vi "getScanValues.vi"(8 "error in (no error)":errorcluster, 11 "ScanCreator in":refnum<class "ScanCreator.lvclass">) -> (0 "error out":errorcluster, 1 "stop":dbl, 2 "start":dbl, 3 "ScanCreator out":refnum<class "ScanCreator.lvclass">, 4 "step":i16)   [LabVIEW 2009, in "Views.lvlib" / "ScriptEditor.lvlib" / "ScanCreator.lvclass"]
uses:
  ScanCreator.lvclass
  ScanCreator.lvclass/ScanCreator.ctl
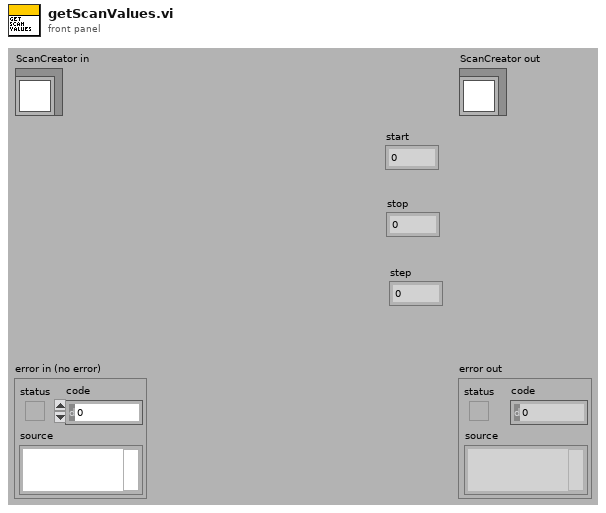
[diagram p1: front panel]
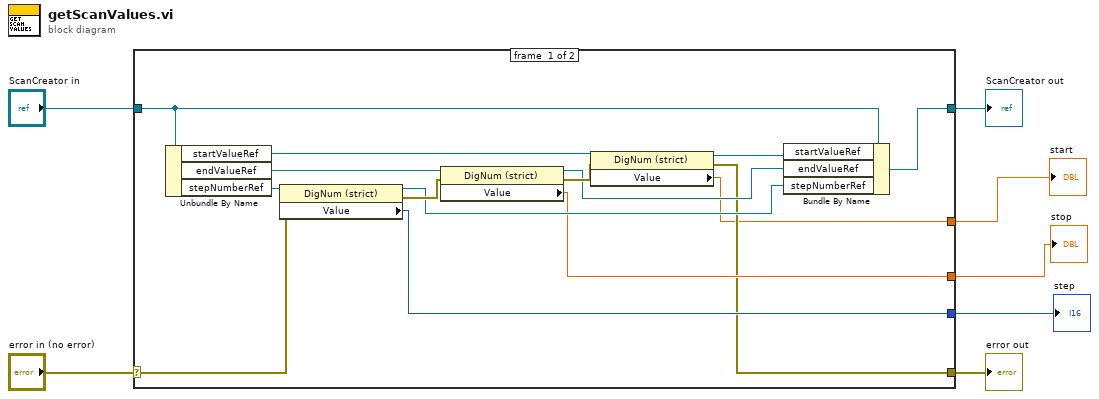
[diagram p0: block diagram]
diagram:
  n1 = case shown="No Error" "error in (no error)" {
    selector: "error in (no error)" -> [w17 w24]
    tunnel: [w11 w24] -> w6
    tunnel: [w8 w23] -> w4
    tunnel: "ScanCreator in" -> [w9 w23]
    tunnel: [w13 _] -> w3
    tunnel: [w12 _] -> w2
    tunnel: [w10 _] -> w1
    frame #0 {
      n2 = Unbundle By Name(w9) -> ("startValueRef"=w20:refnum<vi>, "endValueRef"=w21:refnum<vi>, "stepNumberRef"=w22:refnum<vi>)
      n3 = property class="DigNum (strict)"(reference=w22, error in=w17) -> (reference out=w14:refnum<vi>, error out=w18:errorcluster, "Value"=w13:i16)
      n4 = property class="DigNum (strict)"(reference=w21, error in=w18) -> (reference out=w15:refnum<vi>, error out=w19:errorcluster, "Value"=w12:dbl)
      n5 = property class="DigNum (strict)"(reference=w20, error in=w19) -> (reference out=w16:refnum<vi>, error out=w11:errorcluster, "Value"=w10:dbl)
      n6 = Bundle By Name(cluster=w9, "startValueRef"=w16, "endValueRef"=w15, "stepNumberRef"=w14) -> (w8:refnum<class "ScanCreator.lvclass">)
    }
    frame #1 {
    }
  }
  "error out" <- w6
  "ScanCreator out" <- w4
  "start" <- w1
  "stop" <- w2
  "step" <- w3
